vi "rsidr_core_global.vi"() -> ()   [LabVIEW 2015, in "Rohde&Schwarz CMXP GPRF.lvlib"] (continued)
{"Level"=4, "Class Only"=FALSE, "Identifier"="RSCMXPGPRF_ATTR_SEQUENCER_LIST_ENTRY_DELETE", "Descriptive Name"="Sequencer List Entry Delete", "Data Type"=0, "Command"="SOUR:GPRF:GEN{instance}:SEQ:LIST:ENTR:DEL", "Access"=1, "Range Table"="", "Read Callback"="", "Write Callback"="", "Supported Models"="", "Instrument Options"="", "Flags"=0, "Help"="Deletes the selected entry from the sequencer list.\nAfter the deletion, the selection moves to the next entry, if possible. Otherwise, it moves to the previous entry.\n\nAvailable Repeated Capabilities:\ninstance: i0, i1, i2, i3, i4, i5, i6, i7, i8, i9, i10, i11, i12, i13, i14, i15, i16, i17, i18, i19, i20, i21, i22, i23, i24, i25, i26, i27, i28, i29, i30, i31, i32\r\n\nRemote-control command(s):\nSOURce:GPRF:GEN<i>:SEQuencer:LIST:ENTRy:DELete"}, {"Level"=4, "Class Only"=FALSE, "Identifier"="RSCMXPGPRF_ATTR_SEQUENCER_LIST_ENTRY_MOVE_UP", "Descriptive Name"="Sequencer List Entry Move Up", "Data Type"=0, "Command"="SOUR:GPRF:GEN{instance}:SEQ:LIST:ENTR:MUP", "Access"=1, "Range Table"="", "Read Callback"="", "Write Callback"="", "Supported Models"="", "Instrument Options"="", "Flags"=0, "Help"="Moves the selected entry of the sequencer list one position up.\nThe selection moves with the entry.\n\nAvailable Repeated Capabilities:\ninstance: i0, i1, i2, i3, i4, i5, i6, i7, i8, i9, i10, i11, i12, i13, i14, i15, i16, i17, i18, i19, i20, i21, i22, i23, i24, i25, i26, i27, i28, i29, i30, i31, i32\r\n\nRemote-control command(s):\nSOURce:GPRF:GEN<i>:SEQuencer:LIST:ENTRy:MUP"}, {"Level"=4, "Class Only"=FALSE, "Identifier"="RSCMXPGPRF_ATTR_SEQUENCER_LIST_ENTRY_MOVE_DOWN", "Descriptive Name"="Sequencer List Entry Move Down", "Data Type"=0, "Command"="SOUR:GPRF:GEN{instance}:SEQ:LIST:ENTR:MDOW", "Access"=1, "Range Table"="", "Read Callback"="", "Write Callback"="", "Supported Models"="", "Instrument Options"="", "Flags"=0, "Help"="Moves the selected entry of the sequencer list one position down.\nThe selection moves with the entry.\n\nAvailable Repeated Capabilities:\ninstance: i0, i1, i2, i3, i4, i5, i6, i7, i8, i9, i10, i11, i12, i13, i14, i15, i16, i17, i18, i19, i20, i21, i22, i23, i24, i25, i26, i27, i28, i29, i30, i31, i32\r\n\nRemote-control command(s):\nSOURce:GPRF:GEN<i>:SEQuencer:LIST:ENTRy:MDOWn"}, {"Level"=4, "Class Only"=FALSE, "Identifier"="RSCMXPGPRF_ATTR_SEQUENCER_LIST_ENTRY_CLEAR", "Descriptive Name"="Sequencer List Entry Clear", "Data Type"=4, "Command"="SOUR:GPRF:GEN{instance}:SEQ:LIST:ENTR:CALL", "Access"=1, "Range Table"="", "Read Callback"="", "Write Callback"="", "Supported Models"="", "Instrument Options"="", "Flags"=0, "Help"="Deletes all entries of the sequencer list and creates an entry with default settings.\n\nAvailable Repeated Capabilities:\ninstance: i0, i1, i2, i3, i4, i5, i6, i7, i8, i9, i10, i11, i12, i13, i14, i15, i16, i17, i18, i19, i20, i21, i22, i23, i24, i25, i26, i27, i28, i29, i30, i31, i32\r\n\nRemote-control command(s):\nSOURce:GPRF:GEN<i>:SEQuencer:LIST:ENTRy:CALL"}, {"Level"=4, "Class Only"=FALSE, "Identifier"="RSCMXPGPRF_ATTR_SEQUENCER_LIST_ENTRY_MAX_INDEX", "Descriptive Name"="Sequencer List Entry Max Index", "Data Type"=0, "Command"="SOUR:GPRF:GEN{instance}:SEQ:LIST:MIND?", "Access"=0, "Range Table"="", "Read Callback"="", "Write Callback"="", "Supported Models"="", "Instrument Options"="", "Flags"=0, "Help"="Queries the highest index of the sequencer list. The list contains entries with the indices 0 to <MaximumIndex>.\n\nAvailable Repeated Capabilities:\ninstance: i0, i1, i2, i3, i4, i5, i6, i7, i8, i9, i10, i11, i12, i13, i14, i15, i16, i17, i18, i19, i20, i21, i22, i23, i24, i25, i26, i27, i28, i29, i30, i31, i32\r\n\nRemote-control command(s):\nSOURce:GPRF:GEN<i>:SEQuencer:LIST:MINDex?"}, {"Level"=4, "Class Only"=TRUE, "Identifier"="", "Descriptive Name"="Filling", "Data Type"=0, "Command"="", "Access"=0, "Range Table"="", "Read Callback"="", "Write Callback"="", "Supported Models"="", "Instrument Options"="", "Flags"=0, "Help"="Fill the list"}, {"Level"=5, "Class Only"=FALSE, "Identifier"="RSCMXPGPRF_ATTR_SEQUENCER_LIST_FILLING_START_INDEX", "Descriptive Name"="Sequencer List Filling Start Index", "Data Type"=0, "Command"="SOUR:GPRF:GEN{instance}:SEQ:LIST:FILL:SIND", "Access"=2, "Range Table"="rsCmxpGprf_rngIndex", "Read Callback"="", "Write Callback"="", "Supported Models"="", "Instrument Options"="", "Flags"=0, "Help"="Selects the first index of the sequence to be filled.\nThe maximum value is limited by the index of the highest existing entry plus 1.\n\nAvailable Repeated Capabilities:\ninstance: i0, i1, i2, i3, i4, i5, i6, i7, i8, i9, i10, i11, i12, i13, i14, i15, i16, i17, i18, i19, i20, i21, i22, i23, i24, i25, i26, i27, i28, i29, i30, i31, i32\r\n\nRemote-control command(s):\nSOURce:GPRF:GEN<i>:SEQuencer:LIST:FILL:SINDex"}, {"Level"=5, "Class Only"=FALSE, "Identifier"="RSCMXPGPRF_ATTR_SEQUENCER_LIST_FILLING_RANGE", "Descriptive Name"="Sequencer List Filling Range", "Data Type"=0, "Command"="SOUR:GPRF:GEN{instance}:SEQ:LIST:FILL:RANG", "Access"=2, "Range Table"="rsCmxpGprf_rngListRange", "Read Callback"="", "Write Callback"="", "Supported Models"="", "Instrument Options"="", "Flags"=0, "Help"="Specifies the number of entries to be filled.\nThe maximum is limited by 2000 minus the start index of the sequence.\n\nAvailable Repeated Capabilities:\ninstance: i0, i1, i2, i3, i4, i5, i6, i7, i8, i9, i10, i11, i12, i13, i14, i15, i16, i17, i18, i19, i20, i21, i22, i23, i24, i25, i26, i27, i28, i29, i30, i31, i32\r\n\nRemote-control command(s):\nSOURce:GPRF:GEN<i>:SEQuencer:LIST:FILL:RANGe"}, {"Level"=5, "Class Only"=FALSE, "Identifier"="RSCMXPGPRF_ATTR_SEQUENCER_LIST_FILLING_FREQUENCY_KEEP", "Descriptive Name"="Sequencer List Filling Frequency Keep", "Data Type"=3, "Command"="SOUR:GPRF:GEN{instance}:SEQ:LIST:FILL:FREQ:KEEP", "Access"=2, "Range Table"="", "Read Callback"="", "Write Callback"="", "Supported Models"="", "Instrument Options"="", "Flags"=0, "Help"="Selects whether the frequency of existing entries is kept or overwritten when the sequencer list is filled.\n\nAvailable Repeated Capabilities:\ninstance: i0, i1, i2, i3, i4, i5, i6, i7, i8, i9, i10, i11, i12, i13, i14, i15, i16, i17, i18, i19, i20, i21, i22, i23, i24, i25, i26, i27, i28, i29, i30, i31, i32\r\n\nRemote-control command(s):\nSOURce:GPRF:GEN<i>:SEQuencer:LIST:FILL:FREQuency:KEEP"}, {"Level"=5, "Class Only"=FALSE, "Identifier"="RSCMXPGPRF_ATTR_SEQUENCER_LIST_FILLING_FREQUENCY_START_VALUE", "Descriptive Name"="Sequencer List Filling Frequency Start Value", "Data Type"=1, "Command"="SOUR:GPRF:GEN{instance}:SEQ:LIST:FILL:FREQ:SVAL", "Access"=2, "Range Table"="rsCmxpGprf_rngSpecFreq", "Read Callback"="", "Write Callback"="", "Supported Models"="", "Instrument Options"="", "Flags"=0, "Help"="Configures the start value for filling the sequencer list with frequency values.\n\nAvailable Repeated Capabilities:\ninstance: i0, i1, i2, i3, i4, i5, i6, i7, i8, i9, i10, i11, i12, i13, i14, i15, i16, i17, i18, i19, i20, i21, i22, i23, i24, i25, i26, i27, i28, i29, i30, i31, i32\r\n\nRemote-control command(s):\nSOURce:GPRF:GEN<i>:SEQuencer:LIST:FILL:FREQuency:SVALue"}, {"Level"=5, "Class Only"=FALSE, "Identifier"="RSCMXPGPRF_ATTR_SEQUENCER_LIST_FILLING_FREQUENCY_INCREMENT", "Descriptive Name"="Sequencer List Filling Frequency Increment", "Data Type"=1, "Command"="SOUR:GPRF:GEN{instance}:SEQ:LIST:FILL:FREQ:INCR", "Access"=2, "Range Table"="", "Read Callback"="", "Write Callback"="", "Supported Models"="", "Instrument Options"="", "Flags"=0, "Help"="Configures the increment for filling the sequencer list with frequency values.\n\nAvailable Repeated Capabilities:\ninstance: i0, i1, i2, i3, i4, i5, i6, i7, i8, i9, i10, i11, i12, i13, i14, i15, i16, i17, i18, i19, i20, i21, i22, i23, i24, i25, i26, i27, i28, i29, i30, i31, i32\r\n\nRemote-control command(s):\nSOURce:GPRF:GEN<i>:SEQuencer:LIST:FILL:FREQuency:INCRement"}, {"Level"=5, "Class Only"=FALSE, "Identifier"="RSCMXPGPRF_ATTR_SEQUENCER_LIST_FILLING_DIGITAL_GAIN_START_VALUE", "Descriptive Name"="Sequencer List Filling Digital Gain Start Value", "Data Type"=1, "Command"="SOUR:GPRF:GEN{instance}:SEQ:LIST:FILL:DGA:SVAL", "Access"=2, "Range Table"="rsCmxpGprf_rngDigitalGain", "Read Callback"="", "Write Callback"="", "Supported Models"="", "Instrument Options"="", "Flags"=0, "Help"="Configures the start value for filling the sequencer list with digital gain values.\n\nAvailable Repeated Capabilities:\ninstance: i0, i1, i2, i3, i4, i5, i6, i7, i8, i9, i10, i11, i12, i13, i14, i15, i16, i17, i18, i19, i20, i21, i22, i23, i24, i25, i26, i27, i28, i29, i30, i31, i32\r\n\nRemote-control command(s):\nSOURce:GPRF:GEN<i>:SEQuencer:LIST:FILL:DGAin:SVALue"}, {"Level"=5, "Class Only"=FALSE, "Identifier"="RSCMXPGPRF_ATTR_SEQUENCER_LIST_FILLING_DIGITAL_GAIN_INCREMENT", "Descriptive Name"="Sequencer List Filling Digital Gain Increment", "Data Type"=1, "Command"="SOUR:GPRF:GEN{instance}:SEQ:LIST:FILL:DGA:INCR", "Access"=2, "Range Table"="", "Read Callback"="", "Write Callback"="", "Supported Models"="", "Instrument Options"="", "Flags"=0, "Help"="Configures the increment for filling the sequencer list with digital gain values.\n\nAvailable Repeated Capabilities:\ninstance: i0, i1, i2, i3, i4, i5, i6, i7, i8, i9, i10, i11, i12, i13, i14, i15, i16, i17, i18, i19, i20, i21, i22, i23, i24, i25, i26, i27, i28, i29, i30, i31, i32\r\n\nRemote-control command(s):\nSOURce:GPRF:GEN<i>:SEQuencer:LIST:FILL:DGAin:INCRement"}, {"Level"=5, "Class Only"=FALSE, "Identifier"="RSCMXPGPRF_ATTR_SEQUENCER_LIST_FILLING_DIGITAL_GAIN_KEEP", "Descriptive Name"="Sequencer List Filling Digital Gain Keep", "Data Type"=3, "Command"="SOUR:GPRF:GEN{instance}:SEQ:LIST:FILL:DGA:KEEP", "Access"=2, "Range Table"="", "Read Callback"="", "Write Callback"="", "Supported Models"="", "Instrument Options"="", "Flags"=0, "Help"="Selects whether the digital gain of existing entries is kept or overwritten when the sequencer list is filled.\n\nAvailable Repeated Capabilities:\ninstance: i0, i1, i2, i3, i4, i5, i6, i7, i8, i9, i10, i11, i12, i13, i14, i15, i16, i17, i18, i19, i20, i21, i22, i23, i24, i25, i26, i27, i28, i29, i30, i31, i32\r\n\nRemote-control command(s):\nSOURce:GPRF:GEN<i>:SEQuencer:LIST:FILL:DGAin:KEEP"}, {"Level"=5, "Class Only"=FALSE, "Identifier"="RSCMXPGPRF_ATTR_SEQUENCER_LIST_FILLING_LEVEL_KEEP", "Descriptive Name"="Sequencer List Filling Level Keep", "Data Type"=3, "Command"="SOUR:GPRF:GEN{instance}:SEQ:LIST:FILL:LRMS:KEEP", "Access"=2, "Range Table"="", "Read Callback"="", "Write Callback"="", "Supported Models"="", "Instrument Options"="", "Flags"=0, "Help"="Selects whether the level of existing entries is kept or overwritten when the sequencer list is filled.\n\nAvailable Repeated Capabilities:\ninstance: i0, i1, i2, i3, i4, i5, i6, i7, i8, i9, i10, i11, i12, i13, i14, i15, i16, i17, i18, i19, i20, i21, i22, i23, i24, i25, i26, i27, i28, i29, i30, i31, i32\r\n\nRemote-control command(s):\nSOURce:GPRF:GEN<i>:SEQuencer:LIST:FILL:LRMS:KEEP"}, {"Level"=5, "Class Only"=FALSE, "Identifier"="RSCMXPGPRF_ATTR_SEQUENCER_LIST_FILLING_LEVEL_START_VALUE", "Descriptive Name"="Sequencer List Filling Level Start Value", "Data Type"=1, "Command"="SOUR:GPRF:GEN{instance}:SEQ:LIST:FILL:LRMS:SVAL", "Access"=2, "Range Table"="", "Read Callback"="", "Write Callback"="", "Supported Models"="", "Instrument Options"="", "Flags"=0, "Help"="Configures the start value for filling the sequencer list with level values.\n\nAvailable Repeated Capabilities:\ninstance: i0, i1, i2, i3, i4, i5, i6, i7, i8, i9, i10, i11, i12, i13, i14, i15, i16, i17, i18, i19, i20, i21, i22, i23, i24, i25, i26, i27, i28, i29, i30, i31, i32\r\n\nRemote-control command(s):\nSOURce:GPRF:GEN<i>:SEQuencer:LIST:FILL:LRMS:SVALue"}, {"Level"=5, "Class Only"=FALSE, "Identifier"="RSCMXPGPRF_ATTR_SEQUENCER_LIST_FILLING_LEVEL_INCREMENT", "Descriptive Name"="Sequencer List Filling Level Increment", "Data Type"=1, "Command"="SOUR:GPRF:GEN{instance}:SEQ:LIST:FILL:LRMS:INCR", "Access"=2, "Range Table"="", "Read Callback"="", "Write Callback"="", "Supported Models"="", "Instrument Options"="", "Flags"=0, "Help"="Configures the increment for filling the sequencer list with level values.\n\nAvailable Repeated Capabilities:\ninstance: i0, i1, i2, i3, i4, i5, i6, i7, i8, i9, i10, i11, i12, i13, i14, i15, i16, i17, i18, i19, i20, i21, i22, i23, i24, i25, i26, i27, i28, i29, i30, i31, i32\r\n\nRemote-control command(s):\nSOURce:GPRF:GEN<i>:SEQuencer:LIST:FILL:LRMS:INCRement"}, {"Level"=5, "Class Only"=FALSE, "Identifier"="RSCMXPGPRF_ATTR_SEQUENCER_LIST_FILLING_APPLY", "Descriptive Name"="Sequencer List Filling Apply", "Data Type"=4, "Command"="SOUR:GPRF:GEN{instance}:SEQ:LIST:FILL:APPL", "Access"=1, "Range Table"="", "Read Callback"="", "Write Callback"="", "Supported Models"="", "Instrument Options"="", "Flags"=0, "Help"="Fills the sequencer list with a sequence of entries.\n\nAvailable Repeated Capabilities:\ninstance: i0, i1, i2, i3, i4, i5, i6, i7, i8, i9, i10, i11, i12, i13, i14, i15, i16, i17, i18, i19, i20, i21, i22, i23, i24, i25, i26, i27, i28, i29, i30, i31, i32\r\n\nRemote-control command(s):\nSOURce:GPRF:GEN<i>:SEQuencer:LIST:FILL:APPLy"}, {"Level"=3, "Class Only"=TRUE, "Identifier"="", "Descriptive Name"="Trigger And Marker", "Data Type"=0, "Command"="", "Access"=0, "Range Table"="", "Read Callback"="", "Write Callback"="", "Supported Models"="", "Instrument Options"="", "Flags"=0, "Help"="Trigger and marker settings"}, {"Level"=4, "Class Only"=FALSE, "Identifier"="RSCMXPGPRF_ATTR_SEQUENCER_MARKER_DELAYS", "Descriptive Name"="Sequencer Marker Delays", "Data Type"=6, "Command"="SOUR:GPRF:GEN{instance}:SEQ:MARK:DEL", "Access"=2, "Range Table"="", "Read Callback"="", "Write Callback"="", "Supported Models"="", "Instrument Options"="", "Flags"=0, "Help"="Defines delay times for the ARB output trigger events relative to the marker events.\n\nAvailable Repeated Capabilities:\ninstance: i0, i1, i2, i3, i4, i5, i6, i7, i8, i9, i10, i11, i12, i13, i14, i15, i16, i17, i18, i19, i20, i21, i22, i23, i24, i25, i26, i27, i28, i29, i30, i31, i32\r\n\nRemote-control command(s):\nSOURce:GPRF:GEN<i>:SEQuencer:MARKer:DELays"}, {"Level"=4, "Class Only"=FALSE, "Identifier"="RSCMXPGPRF_ATTR_SEQUENCER_TRIGGER_MANUALLY", "Descriptive Name"="Sequencer Trigger Manually", "Data Type"=4, "Command"="TRIG:GPRF:GEN{instance}:SEQ:MAN:EXEC", "Access"=1, "Range Table"="", "Read Callback"="", "Write Callback"="", "Supported Models"="", "Instrument Options"="", "Flags"=0, "Help"="Triggers the transition to the next sequencer list entry manually.\n\nAvailable Repeated Capabilities:\ninstance: i0, i1, i2, i3, i4, i5, i6, i7, i8, i9, i10, i11, i12, i13, i14, i15, i16, i17, i18, i19, i20, i21, i22, i23, i24, i25, i26, i27, i28, i29, i30, i31, i32\r\n\nRemote-control command(s):\nTRIGger:GPRF:GEN<i>:SEQuencer:MANual:EXECute"}, {"Level"=4, "Class Only"=FALSE, "Identifier"="RSCMXPGPRF_ATTR_SEQUENCER_MEASUREMENT_SOURCE_CATALOG", "Descriptive Name"="Sequencer Measurement Source Catalog", "Data Type"=6, "Command"="TRIG:GPRF:GEN{instance}:SEQ:ISM:CAT?", "Access"=0, "Range Table"="", "Read Callback"="", "Write Callback"="", "Supported Models"="", "Instrument Options"="", "Flags"=0, "Help"="Queries all available measurement source strings.\n\nAvailable Repeated Capabilities:\ninstance: i0, i1, i2, i3, i4, i5, i6, i7, i8, i9, i10, i11, i12, i13, i14, i15, i16, i17, i18, i19, i20, i21, i22, i23, i24, i25, i26, i27, i28, i29, i30, i31, i32\r\n\nRemote-control command(s):\nTRIGger:GPRF:GEN<i>:SEQuencer:ISMeas:CATalog?"}, {"Level"=4, "Class Only"=FALSE, "Identifier"="RSCMXPGPRF_ATTR_SEQUENCER_MEASUREMENT_FOR_TRIGGERING", "Descriptive Name"="Sequencer Measurement For Triggering", "Data Type"=2, "Command"="TRIG:GPRF:GEN{instance}:SEQ:ISM:SOUR", "Access"=2, "Range Table"="", "Read Callback"="", "Write Callback"="", "Supported Models"="", "Instrument Options"="", "Flags"=0, "Help"="Selects a measurement for triggering sequencer list incrementations.\n\nAvailable Repeated Capabilities:\ninstance: i0, i1, i2, i3, i4, i5, i6, i7, i8, i9, i10, i11, i12, i13, i14, i15, i16, i17, i18, i19, i20, i21, i22, i23, i24, i25, i26, i27, i28, i29, i30, i31, i32\r\n\nRemote-control command(s):\nTRIGger:GPRF:GEN<i>:SEQuencer:ISMeas:SOURce"}, {"Level"=4, "Class Only"=FALSE, "Identifier"="RSCMXPGPRF_ATTR_SEQUENCER_TRIGGER_SOURCE_CATALOG", "Descriptive Name"="Sequencer Trigger Source Catalog", "Data Type"=6, "Command"="TRIG:GPRF:GEN{instance}:SEQ:ISTR:CAT?", "Access"=0, "Range Table"="", "Read Callback"="", "Write Callback"="", "Supported Models"="", "Instrument Options"="", "Flags"=0, "Help"="Queries all available trigger source strings.\n\nAvailable Repeated Capabilities:\ninstance: i0, i1, i2, i3, i4, i5, i6, i7, i8, i9, i10, i11, i12, i13, i14, i15, i16, i17, i18, i19, i20, i21, i22, i23, i24, i25, i26, i27, i28, i29, i30, i31, i32\r\n\nRemote-control command(s):\nTRIGger:GPRF:GEN<i>:SEQuencer:ISTRigger:CATalog?"}, {"Level"=4, "Class Only"=FALSE, "Identifier"="RSCMXPGPRF_ATTR_SEQUENCER_SOURCE_FOR_TRIGGERING", "Descriptive Name"="Sequencer Source For Triggering", "Data Type"=2, "Command"="TRIG:GPRF:GEN{instance}:SEQ:ISTR:SOUR", "Access"=2, "Range Table"="", "Read Callback"="", "Write Callback"="", "Supported Models"="", "Instrument Options"="", "Flags"=0, "Help"="Selects a measurement for triggering sequencer list incrementations.\n\nAvailable Repeated Capabilities:\ninstance: i0, i1, i2, i3, i4, i5, i6, i7, i8, i9, i10, i11, i12, i13, i14, i15, i16, i17, i18, i19, i20, i21, i22, i23, i24, i25, i26, i27, i28, i29, i30, i31, i32\r\n\nRemote-control command(s):\nTRIGger:GPRF:GEN<i>:SEQuencer:ISTRigger:SOURce"}, {"Level"=4, "Class Only"=FALSE, "Identifier"="RSCMXPGPRF_ATTR_SEQUENCER_TRIGGER_TIMEOUT", "Descriptive Name"="Sequencer Trigger Timeout", "Data Type"=1, "Command"="TRIG:GPRF:GEN{instance}:SEQ:TOUT", "Access"=2, "Range Table"="rsCmxpGprf_rngSequencerTriggerTimeout", "Read Callback"="", "Write Callback"="", "Supported Models"="", "Instrument Options"="", "Flags"=0, "Help"="Sets a timeout for waiting for a trigger event for List Increment = MEASUREMENT and TRIGGER.\n\nAvailable Repeated Capabilities:\ninstance: i0, i1, i2, i3, i4, i5, i6, i7, i8, i9, i10, i11, i12, i13, i14, i15, i16, i17, i18, i19, i20, i21, i22, i23, i24, i25, i26, i27, i28, i29, i30, i31, i32\r\n\nRemote-control command(s):\nTRIGger:GPRF:GEN<i>:SEQuencer:TOUT"}, {"Level"=1, "Class Only"=TRUE, "Identifier"="", "Descriptive Name"="Analyzer", "Data Type"=0, "Command"="", "Access"=0, "Range Table"="", "Read Callback"="", "Write Callback"="", "Supported Models"="", "Instrument Options"="", "Flags"=0, "Help"="Analyzer configuration."}, {"Level"=2, "Class Only"=FALSE, "Identifier"="RSCMXPGPRF_ATTR_ANALYZER_SCENARIO", "Descriptive Name"="Analyzer Scenario", "Data Type"=0, "Command"="CONF:GPRF:MEAS{instance}:SCEN", "Access"=2, "Range Table"="rsCmxpGprf_rngScenario", "Read Callback"="", "Write Callback"="", "Supported Models"="", "Instrument Options"="", "Flags"=0, "Help"="Selects application scenario.\n\nAvailable Repeated Capabilities:\ninstance: i0, i1, i2, i3, i4, i5, i6, i7, i8, i9, i10, i11, i12, i13, i14, i15, i16, i17, i18, i19, i20, i21, i22, i23, i24, i25, i26, i27, i28, i29, i30, i31, i32\r\n\nRemote-control command(s):\nCONFigure:GPRF:MEAS<i>:SCENario[:ACTivate]"}, {"Level"=2, "Class Only"=FALSE, "Identifier"="RSCMXPGPRF_ATTR_MEASUREMENT_INPUT_CONNECTOR", "Descriptive Name"="Measurement Input Connector", "Data Type"=2, "Command"="ROUT:GPRF:MEAS{instance}:SPAT", "Access"=2, "Range Table"="", "Read Callback"="", "Write Callback"="", "Supported Models"="", "Instrument Options"="", "Flags"=0, "Help"="Selects the input connector for the measured signal.\n\nAvailable Repeated Capabilities:\ninstance: i0, i1, i2, i3, i4, i5, i6, i7, i8, i9, i10, i11, i12, i13, i14, i15, i16, i17, i18, i19, i20, i21, i22, i23, i24, i25, i26, i27, i28, i29, i30, i31, i32\r\n\nRemote-control command(s):\nROUTe:GPRF:MEAS<i>:SPATh"}, {"Level"=2, "Class Only"=FALSE, "Identifier"="RSCMXPGPRF_ATTR_AVAILABLE_SIGNAL_PATHS", "Descriptive Name"="Available Signal Paths", "Data Type"=2, "Command"="CAT:GPRF:MEAS{instance}:SPAT?", "Access"=0, "Range Table"="", "Read Callback"="", "Write Callback"="", "Supported Models"="", "Instrument Options"="", "Flags"=0, "Help"="Returns the names of the available signal paths.\n\nAvailable Repeated Capabilities:\ninstance: i0, i1, i2, i3, i4, i5, i6, i7, i8, i9, i10, i11, i12, i13, i14, i15, i16, i17, i18, i19, i20, i21, i22, i23, i24, i25, i26, i27, i28, i29, i30, i31, i32\r\n\nRemote-control command(s):\nCATalog:GPRF:MEAS<i>:SPATh<stream>?"}, {"Level"=2, "Class Only"=TRUE, "Identifier"="", "Descriptive Name"="RF Settings", "Data Type"=0, "Command"="", "Access"=0, "Range Table"="", "Read Callback"="", "Write Callback"="", "Supported Models"="", "Instrument Options"="", "Flags"=0, "Help"="This class configures the RF input path."}, {"Level"=3, "Class Only"=FALSE, "Identifier"="RSCMXPGPRF_ATTR_ANALYZER_EXPECTED_NOMINAL_POWER", "Descriptive Name"="Analyzer Expected Nominal Power", "Data Type"=1, "Command"="CONF:GPRF:MEAS{instance}:RFS:ENP", "Access"=2, "Range Table"="", "Read Callback"="", "Write Callback"="", "Supported Models"="", "Instrument Options"="", "Flags"=0, "Help"="Sets the expected nominal power of the measured RF signal.\n\nAvailable Repeated Capabilities:\ninstance: i0, i1, i2, i3, i4, i5, i6, i7, i8, i9, i10, i11, i12, i13, i14, i15, i16, i17, i18, i19, i20, i21, i22, i23, i24, i25, i26, i27, i28, i29, i30, i31, i32\r\n\nRemote-control command(s):\nCONFigure:GPRF:MEAS<i>:RFSettings:ENPower"}, {"Level"=3, "Class Only"=FALSE, "Identifier"="RSCMXPGPRF_ATTR_ANALYZER_USER_MARGIN", "Descriptive Name"="Analyzer User Margin", "Data Type"=1, "Command"="CONF:GPRF:MEAS{instance}:RFS:UMAR", "Access"=2, "Range Table"="", "Read Callback"="", "Write Callback"="", "Supported Models"="", "Instrument Options"="", "Flags"=0, "Help"="Sets the margin that the R&S CMW 500 adds to the expected nominal power minus the external input attenuation in order to determine its reference power. The reference power must be within the power range of the selected input connector; refer to the &apos;Specifications&apos;.\n\nAvailable Repeated Capabilities:\ninstance: i0, i1, i2, i3, i4, i5, i6, i7, i8, i9, i10, i11, i12, i13, i14, i15, i16, i17, i18, i19, i20, i21, i22, i23, i24, i25, i26, i27, i28, i29, i30, i31, i32\r\n\nRemote-control command(s):\nCONFigure:GPRF:MEAS<i>:RFSettings:UMARgin"}, {"Level"=3, "Class Only"=FALSE, "Identifier"="RSCMXPGPRF_ATTR_ANALYZER_CENTER_FREQUENCY", "Descriptive Name"="Analyzer Center Frequency", "Data Type"=1, "Command"="CONF:GPRF:MEAS{instance}:RFS:FREQ", "Access"=2, "Range Table"="rsCmxpGprf_rngCenterFrequency", "Read Callback"="", "Write Callback"="", "Supported Models"="", "Instrument Options"="", "Flags"=0, "Help"="Selects the center frequency of the RF analyzer.\n\nAvailable Repeated Capabilities:\ninstance: i0, i1, i2, i3, i4, i5, i6, i7, i8, i9, i10, i11, i12, i13, i14, i15, i16, i17, i18, i19, i20, i21, i22, i23, i24, i25, i26, i27, i28, i29, i30, i31, i32\r\n\nRemote-control command(s):\nCONFigure:GPRF:MEAS<i>:RFSettings:FREQuency"}, {"Level"=2, "Class Only"=TRUE, "Identifier"="", "Descriptive Name"="Routing Settings", "Data Type"=0, "Command"="", "Access"=0, "Range Table"="", "Read Callback"="", "Write Callback"="", "Supported Models"="", "Instrument Options"="", "Flags"=0, "Help"="This class selects the path and connector for the generator and defines an external attenuation value."}, {"Level"=3, "Class Only"=FALSE, "Identifier"="RSCMXPGPRF_ATTR_INPUT_CONNECTOR", "Descriptive Name"="Input Connector", "Data Type"=0, "Command"="ROUT:GPRF:MEAS{instance}:RFS:CONN", "Access"=2, "Range Table"="rsCmxpGprf_rngInputConnector", "Read Callback"="", "Write Callback"="", "Supported Models"="", "Instrument Options"="", "Flags"=0, "Help"="Selects the input connector for the measured RF signal.\n\nAvailable Repeated Capabilities:\ninstance: i0, i1, i2, i3, i4, i5, i6, i7, i8, i9, i10, i11, i12, i13, i14, i15, i16, i17, i18, i19, i20, i21, i22, i23, i24, i25, i26, i27, i28, i29, i30, i31, i32\r\n\nRemote-control command(s):\nROUTe:GPRF:MEAS<i>:RFSettings:CONNector"}, {"Level"=3, "Class Only"=FALSE, "Identifier"="RSCMXPGPRF_ATTR_INPUT_EXTERNAL_ATTENUTATION", "Descriptive Name"="Input External Attenutation", "Data Type"=1, "Command"="CONF:GPRF:MEAS{instance}:RFS:EATT", "Access"=2, "Range Table"="rsCmxpGprf_rngExtAtt", "Read Callback"="", "Write Callback"="", "Supported Models"="", "Instrument Options"="", "Flags"=0, "Help"="Defines an external attenuation (or gain, if the value is negative), to be applied to the selected RF input connector.\n\nAvailable Repeated Capabilities:\ninstance: i0, i1, i2, i3, i4, i5, i6, i7, i8, i9, i10, i11, i12, i13, i14, i15, i16, i17, i18, i19, i20, i21, i22, i23, i24, i25, i26, i27, i28, i29, i30, i31, i32\r\n\nRemote-control command(s):\nCONFigure:GPRF:MEAS<i>:RFSettings:EATTenuation"}, {"Level"=1, "Class Only"=TRUE, "Identifier"="", "Descriptive Name"="Power Measurement", "Data Type"=0, "Command"="", "Access"=0, "Range Table"="", "Read Callback"="", "Write Callback"="", "Supported Models"="", "Instrument Options"="", "Flags"=0, "Help"=""}, {"Level"=2, "Class Only"=TRUE, "Identifier"="", "Descriptive Name"="Configuration", "Data Type"=0, "Command"="", "Access"=0, "Range Table"="", "Read Callback"="", "Write Callback"="", "Supported Models"="", "Instrument Options"="", "Flags"=0, "Help"=""}, {"Level"=3, "Class Only"=FALSE, "Identifier"="RSCMXPGPRF_ATTR_POWER_MEASUREMENT_STEP_LENGTH", "Descriptive Name"="Power Measurement Step Length", "Data Type"=1, "Command"="CONF:GPRF:MEAS{instance}:POW:SLEN", "Access"=2, "Range Table"="rsCmxpGprf_rngStepLength", "Read Callback"="", "Write Callback"="", "Supported Models"="", "Instrument Options"="", "Flags"=0, "Help"="Selects the time between the beginning of two consecutive measured power steps.\n\nAvailable Repeated Capabilities:\ninstance: i0, i1, i2, i3, i4, i5, i6, i7, i8, i9, i10, i11, i12, i13, i14, i15, i16, i17, i18, i19, i20, i21, i22, i23, i24, i25, i26, i27, i28, i29, i30, i31, i32\r\n\nRemote-control command(s):\nCONFigure:GPRF:MEAS<i>:POWer:SLENgth"}, {"Level"=3, "Class Only"=FALSE, "Identifier"="RSCMXPGPRF_ATTR_POWER_MEASUREMENT_MEASUREMENT_LENGTH", "Descriptive Name"="Power Measurement Measurement Length", "Data Type"=1, "Command"="CONF:GPRF:MEAS{instance}:POW:MLEN", "Access"=2, "Range Table"="rsCmxpGprf_rngMeasLength", "Read Callback"="", "Write Callback"="", "Supported Models"="", "Instrument Options"="", "Flags"=0, "Help"="Selects the length of the averaging intervals that the R&S CMW 500 uses to calculate the &apos;Power&apos; results for each measurement step.\n\nAvailable Repeated Capabilities:\ninstance: i0, i1, i2, i3, i4, i5, i6, i7, i8, i9, i10, i11, i12, i13, i14, i15, i16, i17, i18, i19, i20, i21, i22, i23, i24, i25, i26, i27, i28, i29, i30, i31, i32\r\n\nRemote-control command(s):\nCONFigure:GPRF:MEAS<i>:POWer:MLENgth"}, {"Level"=3, "Class Only"=FALSE, "Identifier"="RSCMXPGPRF_ATTR_POWER_MEASUREMENT_REPETITION_MODE", "Descriptive Name"="Power Measurement Repetition Mode", "Data Type"=0, "Command"="CONF:GPRF:MEAS{instance}:POW:REP", "Access"=2, "Range Table"="rsCmxpGprf_rngRepMode", "Read Callback"="", "Write Callback"="", "Supported Models"="", "Instrument Options"="", "Flags"=0, "Help"="Specifies the repetition mode of the measurement; see Statistical Settings. The repetition mode specifies whether the measurement is stopped after a single shot or repeated continuously.\n\nAvailable Repeated Capabilities:\ninstance: i0, i1, i2, i3, i4, i5, i6, i7, i8, i9, i10, i11, i12, i13, i14, i15, i16, i17, i18, i19, i20, i21, i22, i23, i24, i25, i26, i27, i28, i29, i30, i31, i32\r\n\nRemote-control command(s):\nCONFigure:GPRF:MEAS<i>:POWer:REPetition"}, {"Level"=3, "Class Only"=FALSE, "Identifier"="RSCMXPGPRF_ATTR_POWER_MEASUREMENT_COUNT", "Descriptive Name"="Power Measurement Count", "Data Type"=0, "Command"="CONF:GPRF:MEAS{instance}:POW:SCO", "Access"=2, "Range Table"="rsCmxpGprf_rngStatCount", "Read Callback"="", "Write Callback"="", "Supported Models"="", "Instrument Options"="", "Flags"=0, "Help"="Specifies the statistic count of the measurement; see Statistical Settings. The statistic count is equal to the number of measurement intervals per single shot.\n\nAvailable Repeated Capabilities:\ninstance: i0, i1, i2, i3, i4, i5, i6, i7, i8, i9, i10, i11, i12, i13, i14, i15, i16, i17, i18, i19, i20, i21, i22, i23, i24, i25, i26, i27, i28, i29, i30, i31, i32\r\n\nRemote-control command(s):\nCONFigure:GPRF:MEAS<i>:POWer:SCOunt"}, {"Level"=3, "Class Only"=FALSE, "Identifier"="RSCMXPGPRF_ATTR_POWER_MEASUREMENT_FILTER_TYPE", "Descriptive Name"="Power Measurement Filter Type", "Data Type"=0, "Command"="CONF:GPRF:MEAS{instance}:POW:FILT:TYPE", "Access"=2, "Range Table"="rsCmxpGprf_rngPowerMeasFilterType", "Read Callback"="", "Write Callback"="", "Supported Models"="", "Instrument Options"="", "Flags"=0, "Help"="Selects the IF filter type.\n\nAvailable Repeated Capabilities:\ninstance: i0, i1, i2, i3, i4, i5, i6, i7, i8, i9, i10, i11, i12, i13, i14, i15, i16, i17, i18, i19, i20, i21, i22, i23, i24, i25, i26, i27, i28, i29, i30, i31, i32\r\n\nRemote-control command(s):\nCONFigure:GPRF:MEAS<i>:POWer:FILTer:TYPE"}, {"Level"=3, "Class Only"=FALSE, "Identifier"="RSCMXPGPRF_ATTR_POWER_MEASUREMENT_GAUSS_BANDWIDTH", "Descriptive Name"="Power Measurement Gauss Bandwidth", "Data Type"=1, "Command"="CONF:GPRF:MEAS{instance}:POW:FILT:GAUS:BWID", "Access"=2, "Range Table"="rsCmxpGprf_rngGaussBwid", "Read Callback"="", "Write Callback"="", "Supported Models"="", "Instrument Options"="", "Flags"=0, "Help"="Selects the bandwidth for a filter of Gaussian shape.\n\nAvailable Repeated Capabilities:\ninstance: i0, i1, i2, i3, i4, i5, i6, i7, i8, i9, i10, i11, i12, i13, i14, i15, i16, i17, i18, i19, i20, i21, i22, i23, i24, i25, i26, i27, i28, i29, i30, i31, i32\r\n\nRemote-control command(s):\nCONFigure:GPRF:MEAS<i>:POWer:FILTer:GAUSs:BWIDth"}, {"Level"=3, "Class Only"=FALSE, "Identifier"="RSCMXPGPRF_ATTR_POWER_MEASUREMENT_BANDPASS_BANDWIDTH", "Descriptive Name"="Power Measurement Bandpass Bandwidth", "Data Type"=1, "Command"="CONF:GPRF:MEAS{instance}:POW:FILT:BAND:BWID", "Access"=2, "Range Table"="rsCmxpGprf_rngPowerBandpassBandwidth", "Read Callback"="", "Write Callback"="", "Supported Models"="", "Instrument Options"="", "Flags"=0, "Help"="Selects the bandwidth for a filter of Gaussian shape.\n\nAvailable Repeated Capabilities:\ninstance: i0, i1, i2, i3, i4, i5, i6, i7, i8, i9, i10, i11, i12, i13, i14, i15, i16, i17, i18, i19, i20, i21, i22, i23, i24, i25, i26, i27, i28, i29, i30, i31, i32\r\n\nRemote-control command(s):\nCONFigure:GPRF:MEAS<i>:POWer:FILTer:BANDpass:BWIDth"}, {"Level"=3, "Class Only"=FALSE, "Identifier"="RSCMXPGPRF_ATTR_POWER_MEASUREMENT_TIMEOUT", "Descriptive Name"="Power Measurement Timeout", "Data Type"=1, "Command"="CONF:GPRF:MEAS{instance}:POW:TOUT", "Access"=2, "Range Table"="", "Read Callback"="", "Write Callback"="", "Supported Models"="", "Instrument Options"="", "Flags"=0, "Help"="Defines a timeout for the measurement.\n\nAvailable Repeated Capabilities:\ninstance: i0, i1, i2, i3, i4, i5, i6, i7, i8, i9, i10, i11, i12, i13, i14, i15, i16, i17, i18, i19, i20, i21, i22, i23, i24, i25, i26, i27, i28, i29, i30, i31, i32\r\n\nRemote-control command(s):\nCONFigure:GPRF:MEAS<i>:POWer:TOUT"}, {"Level"=3, "Class Only"=FALSE, "Identifier"="RSCMXPGPRF_ATTR_POWER_MEASUREMENT_TRIGGER_SOURCE", "Descriptive Name"="Power Measurement Trigger Source", "Data Type"=2, "Command"="TRIG:GPRF:MEAS{instance}:POW:SOUR", "Access"=2, "Range Table"="", "Read Callback"="", "Write Callback"="", "Supported Models"="", "Instrument Options"="", "Flags"=0, "Help"="Selects the source of the trigger events. Some values are always available in this firmware application. They are listed below. Depending on the installed options additional values may be available. A complete list of all supported values can be displayed using TRIGger:...:CATalog:SOURce?.\n\nAvailable Repeated Capabilities:\ninstance: i0, i1, i2, i3, i4, i5, i6, i7, i8, i9, i10, i11, i12, i13, i14, i15, i16, i17, i18, i19, i20, i21, i22, i23, i24, i25, i26, i27, i28, i29, i30, i31, i32\r\n\nRemote-control command(s):\nTRIGger:GPRF:MEAS<i>:POWer:SOURce"}, {"Level"=3, "Class Only"=FALSE, "Identifier"="RSCMXPGPRF_ATTR_POWER_MEASUREMENT_TRIGGER_SLOPE", "Descriptive Name"="Power Measurement Trigger Slope", "Data Type"=0, "Command"="TRIG:GPRF:MEAS{instance}:POW:SLOP", "Access"=2, "Range Table"="rsCmxpGprf_rngTrigSlope", "Read Callback"="", "Write Callback"="", "Supported Models"="", "Instrument Options"="", "Flags"=0, "Help"="Qualifies whether the trigger event is generated at the rising or at the falling edge of the trigger pulse (valid for the power trigger sources.\n\nAvailable Repeated Capabilities:\ninstance: i0, i1, i2, i3, i4, i5, i6, i7, i8, i9, i10, i11, i12, i13, i14, i15, i16, i17, i18, i19, i20, i21, i22, i23, i24, i25, i26, i27, i28, i29, i30, i31, i32\r\n\nRemote-control command(s):\nTRIGger:GPRF:MEAS<i>:POWer:SLOPe"}, {"Level"=3, "Class Only"=FALSE, "Identifier"="RSCMXPGPRF_ATTR_POWER_MEASUREMENT_TRIGGER_THRESHOLD", "Descriptive Name"="Power Measurement Trigger Threshold", "Data Type"=1, "Command"="TRIG:GPRF:MEAS{instance}:POW:THR", "Access"=2, "Range Table"="rsCmxpGprf_rngTrigThreshold", "Read Callback"="", "Write Callback"="", "Supported Models"="", "Instrument Options"="", "Flags"=0, "Help"="Defines the trigger threshold for the power trigger sources.\n\nAvailable Repeated Capabilities:\ninstance: i0, i1, i2, i3, i4, i5, i6, i7, i8, i9, i10, i11, i12, i13, i14, i15, i16, i17, i18, i19, i20, i21, i22, i23, i24, i25, i26, i27, i28, i29, i30, i31, i32\r\n\nRemote-control command(s):\nTRIGger:GPRF:MEAS<i>:POWer:THReshold"}, {"Level"=3, "Class Only"=FALSE, "Identifier"="RSCMXPGPRF_ATTR_POWER_MEASUREMENT_TRIGGER_OFFSET", "Descriptive Name"="Power Measurement Trigger Offset", "Data Type"=1, "Command"="TRIG:GPRF:MEAS{instance}:POW:OFFS", "Access"=2, "Range Table"="rsCmxpGprf_rngTrigOffsetIFPow", "Read Callback"="", "Write Callback"="", "Supported Models"="", "Instrument Options"="", "Flags"=0, "Help"="Defines a delay time for the Internal Trigger (Internal). The trigger offset delays the start of the measurement relative to the trigger event.\n\nAvailable Repeated Capabilities:\ninstance: i0, i1, i2, i3, i4, i5, i6, i7, i8, i9, i10, i11, i12, i13, i14, i15, i16, i17, i18, i19, i20, i21, i22, i23, i24, i25, i26, i27, i28, i29, i30, i31, i32\r\n\nRemote-control command(s):\nTRIGger:GPRF:MEAS<i>:POWer:OFFSet"}, {"Level"=3, "Class Only"=FALSE, "Identifier"="RSCMXPGPRF_ATTR_POWER_MEASUREMENT_TRIGGER_TIMEOUT", "Descriptive Name"="Power Measurement Trigger Timeout", "Data Type"=1, "Command"="TRIG:GPRF:MEAS{instance}:POW:TOUT", "Access"=2, "Range Table"="rsCmxpGprf_rngTrigTout", "Read Callback"="", "Write Callback"="", "Supported Models"="", "Instrument Options"="", "Flags"=0, "Help"="Sets a time after which the initiated measurement is automatically terminated if it does not receive a trigger event.\n\nAvailable Repeated Capabilities:\ninstance: i0, i1, i2, i3, i4, i5, i6, i7, i8, i9, i10, i11, i12, i13, i14, i15, i16, i17, i18, i19, i20, i21, i22, i23, i24, i25, i26, i27, i28, i29, i30, i31, i32\r\n\nRemote-control command(s):\nTRIGger:GPRF:MEAS<i>:POWer:TOUT"}, {"Level"=3, "Class Only"=FALSE, "Identifier"="RSCMXPGPRF_ATTR_POWER_MEASUREMENT_TRIGGER_TIMEOUT_ENABLED", "Descriptive Name"="Power Measurement Trigger Timeout Enabled", "Data Type"=3, "Command"="TRIG:GPRF:MEAS{instance}:POW:TOUT", "Access"=2, "Range Table"="", "Read Callback"="", "Write Callback"="", "Supported Models"="", "Instrument Options"="", "Flags"=0, "Help"="Disables timeout | enables timeout using the previous/default values.\n\nAvailable Repeated Capabilities:\ninstance: i0, i1, i2, i3, i4, i5, i6, i7, i8, i9, i10, i11, i12, i13, i14, i15, i16, i17, i18, i19, i20, i21, i22, i23, i24, i25, i26, i27, i28, i29, i30, i31, i32\r\n\nRemote-control command(s):\nTRIGger:GPRF:MEAS<i>:POWer:TOUT"}, {"Level"=3, "Class Only"=FALSE, "Identifier"="RSCMXPGPRF_ATTR_POWER_MEASUREMENT_TRIGGER_CATALOG", "Descriptive Name"="Power Measurement Trigger Catalog", "Data Type"=2, "Command"="TRIG:GPRF:MEAS{instance}:POW:CAT:SOUR?", "Access"=0, "Range Table"="", "Read Callback"="", "Write Callback"="", "Supported Models"="", "Instrument Options"="", "Flags"=0, "Help"="Lists all trigger source values that can be set using TRIGger:GPRF:MEAS<i>:POWer:SOURce.\n\nAvailable Repeated Capabilities:\ninstance: i0, i1, i2, i3, i4, i5, i6, i7, i8, i9, i10, i11, i12, i13, i14, i15, i16, i17, i18, i19, i20, i21, i22, i23, i24, i25, i26, i27, i28, i29, i30, i31, i32\r\n\nRemote-control command(s):\nTRIGger:GPRF:MEAS<i>:POWer:CATalog:SOURce?"}, {"Level"=3, "Class Only"=FALSE, "Identifier"="RSCMXPGPRF_ATTR_POWER_MEASUREMENT_TRIGGER_MODE", "Descriptive Name"="Power Measurement Trigger Mode", "Data Type"=0, "Command"="TRIG:GPRF:MEAS{instance}:POW:MODE", "Access"=2, "Range Table"="rsCmxpGprf_rngTrigMode", "Read Callback"="", "Write Callback"="", "Supported Models"="", "Instrument Options"="", "Flags"=0, "Help"="Selects the measurement sequence that is triggered by each single trigger event. This setting is not valid for free run measurements.\n\nAvailable Repeated Capabilities:\ninstance: i0, i1, i2, i3, i4, i5, i6, i7, i8, i9, i10, i11, i12, i13, i14, i15, i16, i17, i18, i19, i20, i21, i22, i23, i24, i25, i26, i27, i28, i29, i30, i31, i32\r\n\nRemote-control command(s):\nTRIGger:GPRF:MEAS<i>:POWer:MODE"}, {"Level"=3, "Class Only"=FALSE, "Identifier"="RSCMXPGPRF_ATTR_POWER_MEASUREMENT_TRIGGER_GAP", "Descriptive Name"="Power Measurement Trigger Gap", "Data Type"=1, "Command"="TRIG:GPRF:MEAS{instance}:POW:MGAP", "Access"=2, "Range Table"="rsCmxpGprf_rngTriggerGap", "Read Callback"="", "Write Callback"="", "Supported Models"="", "Instrument Options"="", "Flags"=0, "Help"="Defines a minimum duration of the power-down periods (gaps) between two triggered IF power pulses.\n\nAvailable Repeated Capabilities:\ninstance: i0, i1, i2, i3, i4, i5, i6, i7, i8, i9, i10, i11, i12, i13, i14, i15, i16, i17, i18, i19, i20, i21, i22, i23, i24, i25, i26, i27, i28, i29, i30, i31, i32\r\n\nRemote-control command(s):\nTRIGger:GPRF:MEAS<i>:POWer:MGAP"}, {"Level"=3, "Class Only"=FALSE, "Identifier"="RSCMXPGPRF_ATTR_POWER_MEASUREMENT_LIST_MODE_STATE", "Descriptive Name"="Power Measurement List Mode State", "Data Type"=3, "Command"="CONF:GPRF:MEAS{instance}:POW:LIST", "Access"=2, "Range Table"="", "Read Callback"="", "Write Callback"="", "Supported Models"="", "Instrument Options"="", "Flags"=0, "Help"="Selects the sequence mode of the &apos;Power&apos; measurement.\n\nAvailable Repeated Capabilities:\ninstance: i0, i1, i2, i3, i4, i5, i6, i7, i8, i9, i10, i11, i12, i13, i14, i15, i16, i17, i18, i19, i20, i21, i22, i23, i24, i25, i26, i27, i28, i29, i30, i31, i32\r\n\nRemote-control command(s):\nCONFigure:GPRF:MEAS<i>:POWer:LIST"}, {"Level"=3, "Class Only"=FALSE, "Identifier"="RSCMXPGPRF_ATTR_POWER_MEASUREMENT_LIST_RESULTS_COUNT", "Descriptive Name"="Power Measurement List Results Count", "Data Type"=0, "Command"="CONF:GPRF:MEAS{instance}:POW:LIST:COUN?", "Access"=0, "Range Table"="", "Read Callback"="", "Write Callback"="", "Supported Models"="", "Instrument Options"="", "Flags"=0, "Help"="Queries the total number of results, depending on the sequence mode.\n\nAvailable Repeated Capabilities:\ninstance: i0, i1, i2, i3, i4, i5, i6, i7, i8, i9, i10, i11, i12, i13, i14, i15, i16, i17, i18, i19, i20, i21, i22, i23, i24, i25, i26, i27, i28, i29, i30, i31, i32\r\n\nRemote-control command(s):\nCONFigure:GPRF:MEAS<i>:POWer:LIST:COUNt?"}, {"Level"=3, "Class Only"=FALSE, "Identifier"="RSCMXPGPRF_ATTR_POWER_MEASUREMENT_LIST_START", "Descriptive Name"="Power Measurement List Start", "Data Type"=0, "Command"="CONF:GPRF:MEAS{instance}:POW:LIST:STAR", 
